vi "Difference Quotient.vi"(3 "X":dbl[](array[numeric]), 4 "Y":dbl[](array[numeric])) -> (1 "dY/dX":dbl[](array[numeric]))   [LabVIEW 2010]
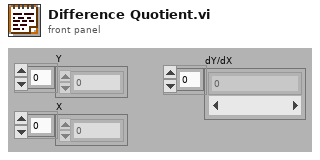
[diagram p1: front panel]
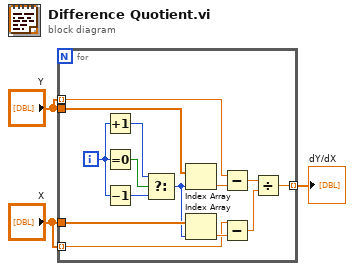
[diagram p0: block diagram]
diagram:
  n1 = for {
    tunnel: "Y" -> [w13]
    tunnel: "X" -> [w10]
    tunnel: [w6] -> w3 mode=indexing
    tunnel: "Y" -> [w5] mode=indexing
    tunnel: "X" -> [w4] mode=indexing
    i -> [w16]
    n2 = Increment(x=w16) -> (x+1=w15:i32)
    n3 = Equal To 0?(x=w16) -> (x = 0?=w17:bool)
    n4 = Decrement(x=w16) -> (x-1=w14:i32)
    n5 = Select(t=w15, s=w17, f=w14) -> (s? t:f=w9:i32)
    n6 = Index Array(array=w13, index=w9) -> (element=w12:dbl)
    n7 = Index Array(array=w10, index=w9) -> (element=w8:dbl)
    n8 = Subtract(x=w5, y=w12) -> (x-y=w11:dbl)
    n9 = Subtract(x=w4, y=w8) -> (x-y=w7:dbl)
    n10 = Divide(x=w11, y=w7) -> (x/y=w6:dbl)
  }
  "dY/dX" <- w3
